vi "Format Into File and Scan From File.vi"() -> ()   [LabVIEW 2023]
doc: "This example shows how the Format Into File and Scan From File functions operate using different options."
panel:
  in  "Operation":u16(ring) items=["Input File as Path", "Input File as Refnum", "Specifying a Format String"]
  in  "Format String":string="Path Value - %s\nString Value - %s\nBoolean Value - %s\nNumeric Value - %d\nTimestamp Value - %T"
  out "Write Time":timestamp
  in  "Write Numeric":i32=12345
  in  "Write Boolean":bool
  in  "Write String":string="sample_string"
  in  "Write Path":path=path "C:/sample_path/subfolder"
  out "Read Time":timestamp
  out "Read Numeric":i32
  out "Read Boolean":bool
  out "Read String":string
  out "Read Path":path
  # "Overview: Demonstrates the use of the Format Into File function to write data to a text file, and the Scan From File function to read data from that text file.\nInstructions:\n1. Specify an Operation to illustrate a particular use case for the Format Into File and Scan From File functions.\n2. Run the VI. The 'Write' values below will be written to the file, then read back and displayed in the 'Read' values.\n3. Delete the text file (located at [LabVIEW Data]\\Example Format Scan File.txt) when you are done."
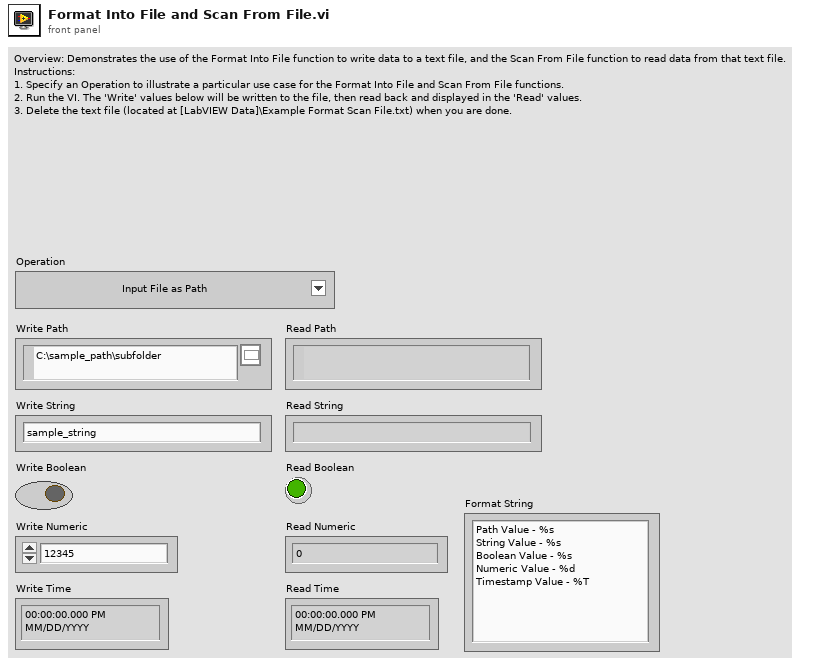
[diagram p1: front panel]
types:
  T1 = enum16{"open", "replace", "create", "open or create", "replace or create", "replace or create with confirmation"}
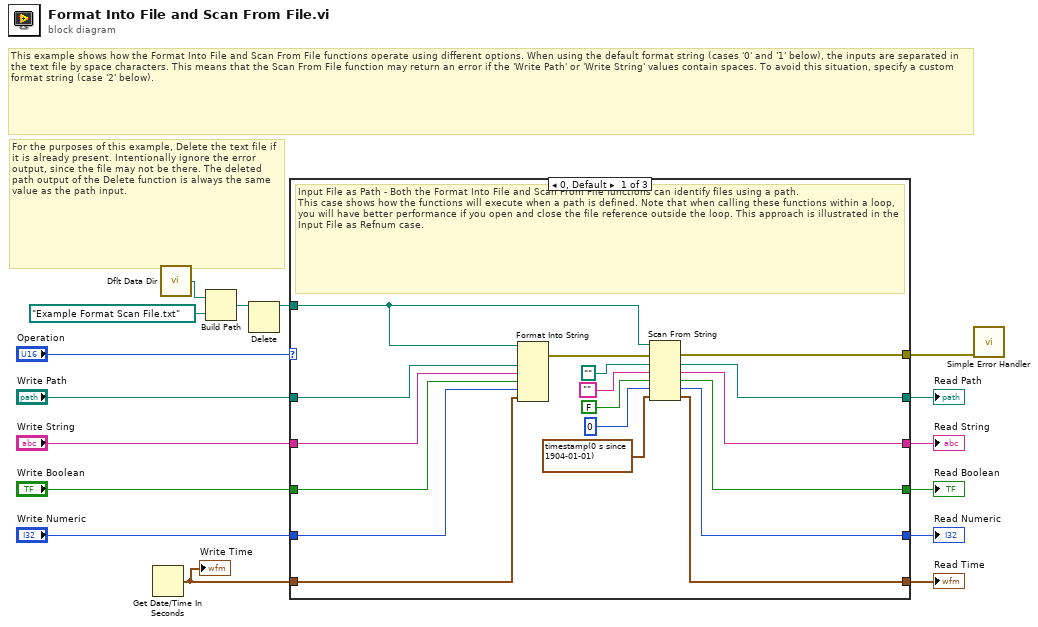
[diagram p0: block diagram]
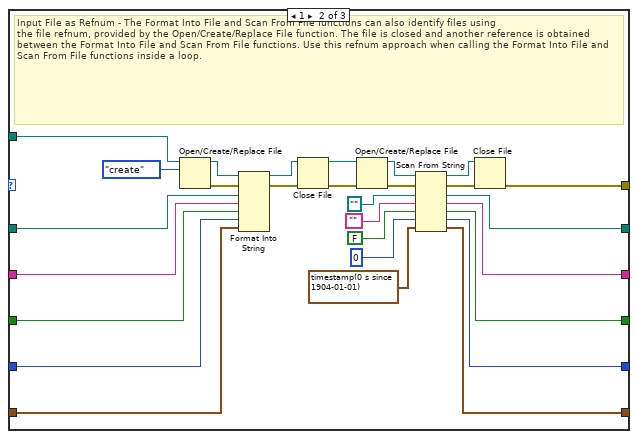
[diagram p2: hidden frame]
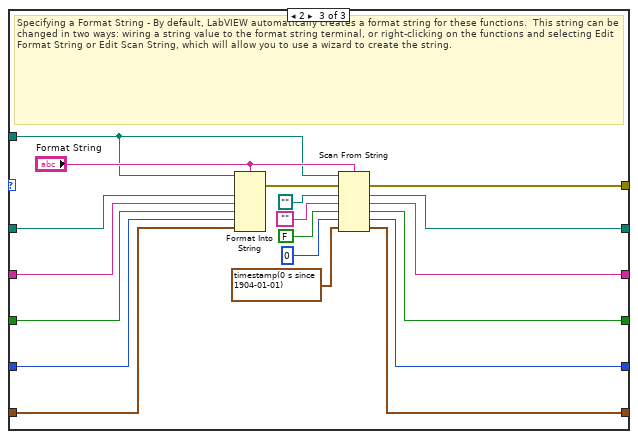
[diagram p3: hidden frame]
diagram:
  # "For the purposes of this example, Delete the text file if it is already present. Intentionally ignore the error output, since the file may not be there. The deleted path output of the Delete function is always the same value as the path input."
  # "This example shows how the Format Into File and Scan From File functions operate using different options. When using the default format string (cases '0' and '1' below), the inputs are separated in the text file by space characters. This means that the Scan From File function may return an error if the 'Write Path' or 'Write String' values contain spaces. To avoid this situation, specify a custom format string (case '2' below)."
  n1 = Get Date/Time In Seconds() -> (seconds since 1Jan1904=w12:timestamp)
  "Write Time" <- w12
  n2 = call <vilib>:"Dflt Data Dir.vi"() -> ("App:Default Data Directory"=w3:path)
  n3 = Build Path(base path=w3, name or relative path=path "Example Format Scan File.txt" ("default name")) -> (appended path=w5:path)
  n4 = Delete(path (use dialog)=w5) -> (deleted path=w2:path)  [unwired: 4 in, 2 out]
  n5 = case shown="0, Default" "Operation" {
    tunnel: [w33 w53 w79] -> w1
    tunnel: "Write Path" -> [w32 w51 w78]
    tunnel: "Write String" -> [w31 w50 w77]
    tunnel: "Write Boolean" -> [w30 w49 w76]
    tunnel: "Write Numeric" -> [w29 w48 w75]
    tunnel: w12 -> [w24 w47 w74]
    tunnel: [w22 w37 w68] -> w11
    tunnel: [w21 w38 w67] -> w10
    tunnel: [w20 w39 w66] -> w9
    tunnel: [w19 w40 w65] -> w8
    tunnel: [w18 w41 w64] -> w7
    tunnel: w2 -> [w17 w36 w63]
    frame 0, Default {
      # "Input File as Path - Both the Format Into File and Scan From File functions can identify files using a path.  \nThis case shows how the functions will execute when a path is defined. Note that when calling these functions within a loop, you will have better performance if you open and close the file reference outside the loop. This approach is illustrated in the Input File as Refnum case."
      n6 = Format Into String(initial string=w17, w32, w31, w30, w29, w24) -> (error out=w34:errorcluster)  [unwired: 2 in, 1 out]
      n7 = Scan From String(w17, w34, default 1=path "", default 2="", default 3=FALSE, default 4=0, default 5=timestamp(0 s since 1904-01-01) ("seconds since 1Jan1904")) -> (w33:errorcluster, output 1=w22:path, output 2=w21:string, output 3=w20:bool, output 4=w19:i32, output 5=w18:timestamp)  [unwired: 1 in, 1 out]
    }
    frame 1 {
      # "Input File as Refnum - The Format Into File and Scan From File functions can also identify files using \nthe file refnum, provided by the Open/Create/Replace File function. The file is closed and another reference is obtained between the Format Into File and Scan From File functions. Use this refnum approach when calling the Format Into File and Scan From File functions inside a loop."
      n8 = Open/Create/Replace File(file path (use dialog)=w36, operation (0:open)=T1."create") -> (refnum out=w61:refnum<file>, error out=w55:errorcluster)  [unwired: 1 in, 4 out]
      n9 = Format Into String(initial string=w61, error in=w55, w51, w50, w49, w48, w47) -> (resulting string=w60:refnum<file>, error out=w56:errorcluster)  [unwired: 1 in]
      n10 = Close File(refnum=w60, error in=w56) -> (path=w59:path, error out=w58:errorcluster)
      n11 = Open/Create/Replace File(file path (use dialog)=w59, error in=w58) -> (refnum out=w35:refnum<file>, error out=w52:errorcluster)  [unwired: 5 out]
      n12 = Scan From String(w35, w52, default 1=path "", default 2="", default 3=FALSE, default 4=0, default 5=timestamp(0 s since 1904-01-01) ("seconds since 1Jan1904")) -> (w57:refnum<file>, w54:errorcluster, output 1=w37:path, output 2=w38:string, output 3=w39:bool, output 4=w40:i32, output 5=w41:timestamp)  [unwired: 1 in]
      n13 = Close File(refnum=w57, error in=w54) -> (error out=w53:errorcluster)  [unwired: 1 out]
    }
    frame 2 {
      # "Specifying a Format String - By default, LabVIEW automatically creates a format string for these functions.  This string can be changed in two ways: wiring a string value to the format string terminal, or right-clicking on the functions and selecting Edit Format String or Edit Scan String, which will allow you to use a wizard to create the string."
      n14 = Format Into String(format string="Format String", initial string=w63, w78, w77, w76, w75, w74) -> (error out=w80:errorcluster)  [unwired: 1 in, 1 out]
      n15 = Scan From String("Format String", w63, w80, default 1=path "", default 2="", default 3=FALSE, default 4=0, default 5=timestamp(0 s since 1904-01-01) ("seconds since 1Jan1904")) -> (w79:errorcluster, output 1=w68:path, output 2=w67:string, output 3=w66:bool, output 4=w65:i32, output 5=w64:timestamp)  [unwired: 1 out]
    }
  }
  "Read Path" <- w11
  "Read String" <- w10
  "Read Boolean" <- w9
  "Read Numeric" <- w8
  "Read Time" <- w7
  n16 = call <vilib>:"Simple Error Handler.vi"("error in (no error)"=w1) -> ()  [unwired: 1 in, 8 out]
